vi "action.vi"(0 "HGF_FGV_Size":refnum<class "HGF_FGV_Size.lvclass">, 2 "Objects":refnum<class>[](array[class]), 5 "error in (no error)":errorcluster) -> (14 "dup HGF_FGV_Size":refnum<class "HGF_FGV_Size.lvclass">, 16 "dup Objects":refnum<class>[](array[class]), 19 "error out":errorcluster)   [LabVIEW 2012, in "HGF_FGV.lvlib" / "HGF_FGV_Size.lvclass"]
doc: "This is a dynamic dispatch VI. It must be overwritten by child classes.to implement the concrete action."
uses:
  HGF_FGV_Size.lvclass
  HGF_FGV_Size.lvclass/HGF_FGV_Size.ctl
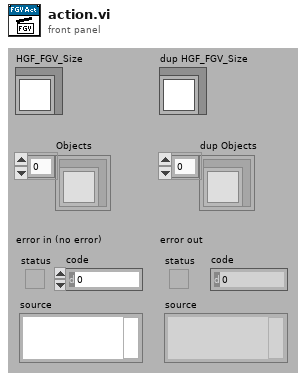
[diagram p1: front panel]
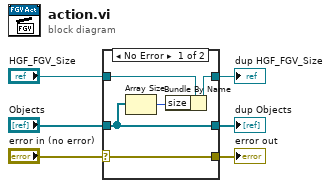
[diagram p0: block diagram]
diagram:
  n1 = case shown="No Error" "error in (no error)" {
    selector: "error in (no error)" -> [w11 w14]
    tunnel: [w11 w14] -> w5
    tunnel: [w9 w13] -> w3
    tunnel: "HGF_FGV_Size" -> [w10 w13]
    tunnel: [w8 w12] -> w2
    tunnel: "Objects" -> [w8 w12]
    frame No Error {
      n2 = Array Size(array=w8) -> (size(s)=w7:i32)
      n3 = Bundle By Name(cluster=w10, "size"=w7) -> (w9:refnum<class "HGF_FGV_Size.lvclass">)
    }
    frame Error {
    }
  }
  "error out" <- w5
  "dup HGF_FGV_Size" <- w3
  "dup Objects" <- w2
